vi "APC_9056_FPGA_main.vi"() -> ()   [LabVIEW 2020]
uses:
  <vilib>/Platform/TimedLoop/XDataNode/timing_clust.ctl
  <vilib>/Platform/TimedLoop/XDataNode/nitl_modes.ctl
  <vilib>/Platform/TimedLoop/XDataNode/wakeup.ctl
  <vilib>/rvi/eio/common/nirviEmuTemplateMethod_errors.vi
  <vilib>/rvi/Emulation/niFpgaGetClockAttributes.vi
  <vilib>/rvi/Emulation/niFpgaSctlEmulationGetInTimedLoop.vi
  <vilib>/rvi/Emulation/niFpgaEmulationReportErrorSimple.vi
  <vilib>/rvi/Emulation/niFpgaCriticalErrorInLSC.vi
  <vilib>/rvi/Emulation/niFpgaProcessEmulError.vi
  <vilib>/eio/EIONode/EIONode.xnode
  <vilib>/platform/TimedLoop/XDataNode/XDataNode.xnode
  <vilib>/Platform/TimedLoop/XDataNode/XDNodeRunTimeDep.lvlib
panel:
  out "counter":u32
  in  "margin":u32=250
  in  "Ticks per toggle":u32[](array[numeric])=[13000, 12000, 11000, 10000, 9000, 8000, 7000, 6000, 5000, 4000, 3000, 2000, 1000]
  out "Detected mode":i16
  out "RT counter overflow: setting SAFE mode":bool
  in  "Counter max [10 ms clock]":u32=100
  out "Watchdog counter":u32
  in  "RT watchdog":bool
  out "NI9375/DI15":bool
  out "NI9375/DI14":bool
  out "NI9375/DI13":bool
  out "NI9375/DI12":bool
  out "NI9375/DI11":bool
  out "NI9375/DI10":bool
  out "NI9375/DI9":bool
  out "NI9375/DI8":bool
  out "NI9375/DI7":bool
  out "NI9375/DI6":bool
  out "NI9375/DI5":bool
  out "NI9375/DI4":bool
  out "NI9375/DI3":bool
  out "NI9375/DI2":bool
  out "NI9375/DI1":bool
  out "NI9375/DI0":bool
  in  "NI9375/DO15":bool
  in  "NI9375/DO14":bool
  in  "NI9375/DO13":bool
  in  "NI9375/DO12":bool
  in  "NI9375/DO11":bool
  in  "NI9375/DO10":bool
  in  "NI9375/DO9":bool
  in  "NI9375/DO8":bool
  in  "NI9375/DO7":bool
  in  "NI9375/DO6":bool
  in  "NI9375/DO5":bool
  in  "NI9375/DO4":bool
  in  "NI9375/DO3":bool
  in  "NI9375/DO2":bool
  in  "NI9375/DO1":bool
  in  "NI9375/DO0":bool
  in  "NI9266/AO7":fxp<+,20,-5>
  in  "NI9266/AO6":fxp<+,20,-5>
  in  "NI9266/AO5":fxp<+,20,-5>
  in  "NI9266/AO4":fxp<+,20,-5>
  in  "NI9266/AO3":fxp<+,20,-5>
  in  "NI9266/AO2":fxp<+,20,-5>
  in  "NI9266/AO1":fxp<+,20,-5>
  in  "NI9266/AO0":fxp<+,20,-5>
  in  "NI9264/AO15":fxp<+/-,20,5>
  in  "NI9264/AO14":fxp<+/-,20,5>
  in  "NI9264/AO13":fxp<+/-,20,5>
  in  "NI9264/AO12":fxp<+/-,20,5>
  in  "NI9264/AO11":fxp<+/-,20,5>
  in  "NI9264/AO10":fxp<+/-,20,5>
  in  "NI9264/AO9":fxp<+/-,20,5>
  in  "NI9264/AO8":fxp<+/-,20,5>
  in  "NI9264/AO7":fxp<+/-,20,5>
  in  "NI9264/AO6":fxp<+/-,20,5>
  in  "NI9264/AO5":fxp<+/-,20,5>
  in  "NI9264/AO4":fxp<+/-,20,5>
  in  "NI9264/AO3":fxp<+/-,20,5>
  in  "NI9264/AO2":fxp<+/-,20,5>
  in  "NI9264/AO1":fxp<+/-,20,5>
  in  "NI9264/AO0":fxp<+/-,20,5>
  out "dT HB (ms)":u32
  out "dT inj (ticks)":u32
  out "FPGA Hearbeat":bool
  out "Chassis Temp Raw (x4 C)":i16=143
  # "This is low level FPGA interface only! \nDO NOT USE DIRECTLY\nUse RT module to configure"
  # "NI9264 interface"
  # "General Monitoring & Control"
  # "NI9266 interface"
  # "USER LED1 is also \nbroadcasting the \nhearbeat at 1Hz"
  # "NI9375 interface"
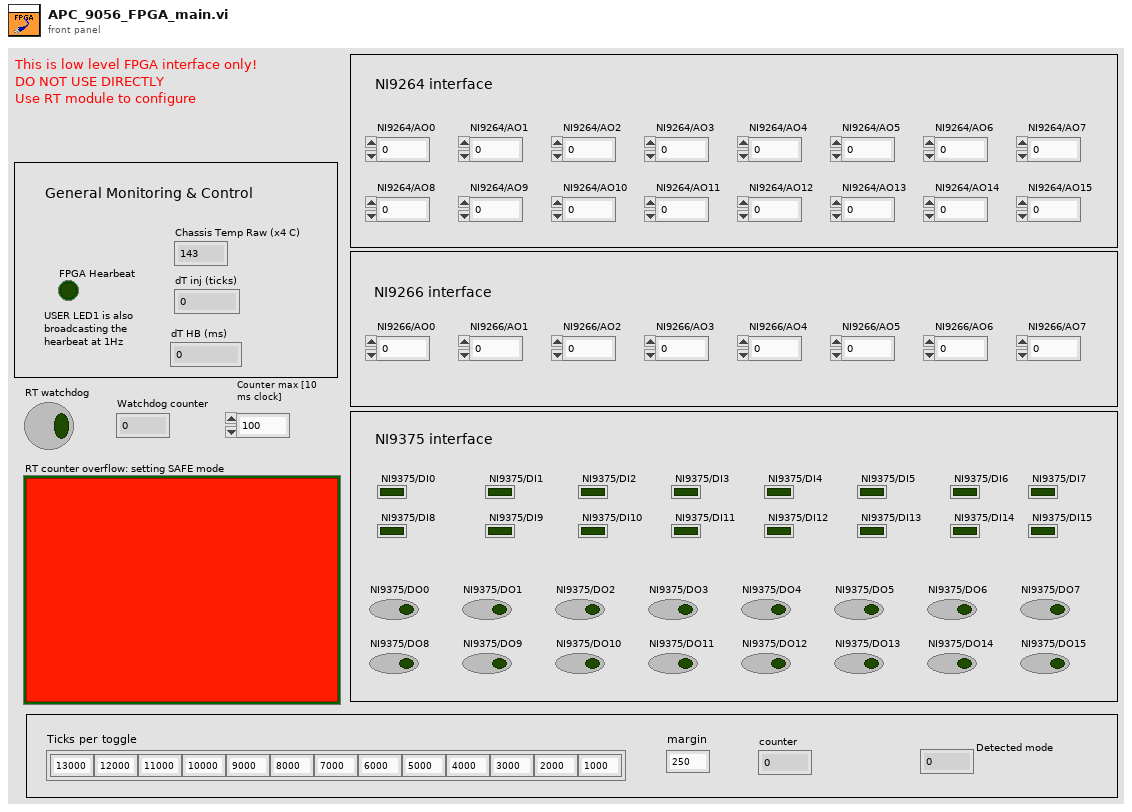
[diagram p1: front panel]
types:
  T1 = typedef "XDNodeRunTimeDep.lvlib/timing_clust.ctl" = cluster{"Expected End [f-1]":u64, "Actual End [f-1]":u64, "Finished Late? [f-1]":bool, "Expected End [i-1]":u64, "Actual End [i-1]":u64, "Finished Late? [i-1]":bool, "Expected Start [i]":u64, "Actual Start [i]":u64, "Expected Start [f]":u64, "Actual Start [f]":u64, "Source Name":string, "Structure Name":string, "Period":i64, "Deadline":i64, "Offset":i64, "Start":i64, "Priority":i32, "Timeout":i32, "Mode":T2, "Wakeup Reason":T3, "Error":errorcluster, "Source Type":string, "Secondary Source Type":string, "Global End Time":u64, "Global Start Time":u64, "Frame Duration":u64, "Iteration Duration":u64, "Assigned CPU":i32, "I/O Scan Engine Mode":u32}
  T2 = typedef "XDNodeRunTimeDep.lvlib/nitl_modes.ctl" = enum32{"No Change", "Process missed periods, maintain original phase", "Discard missed periods, maintain original phase", "Process missed periods, ignore original phase", "Discard missed periods, ignore original phase"}
  T3 = typedef "XDNodeRunTimeDep.lvlib/wakeup.ctl" = enum32{"Normal", "Aborted", "Asynchronous wakeup", "Timing source error", "Timed loop error", "Timeout"}
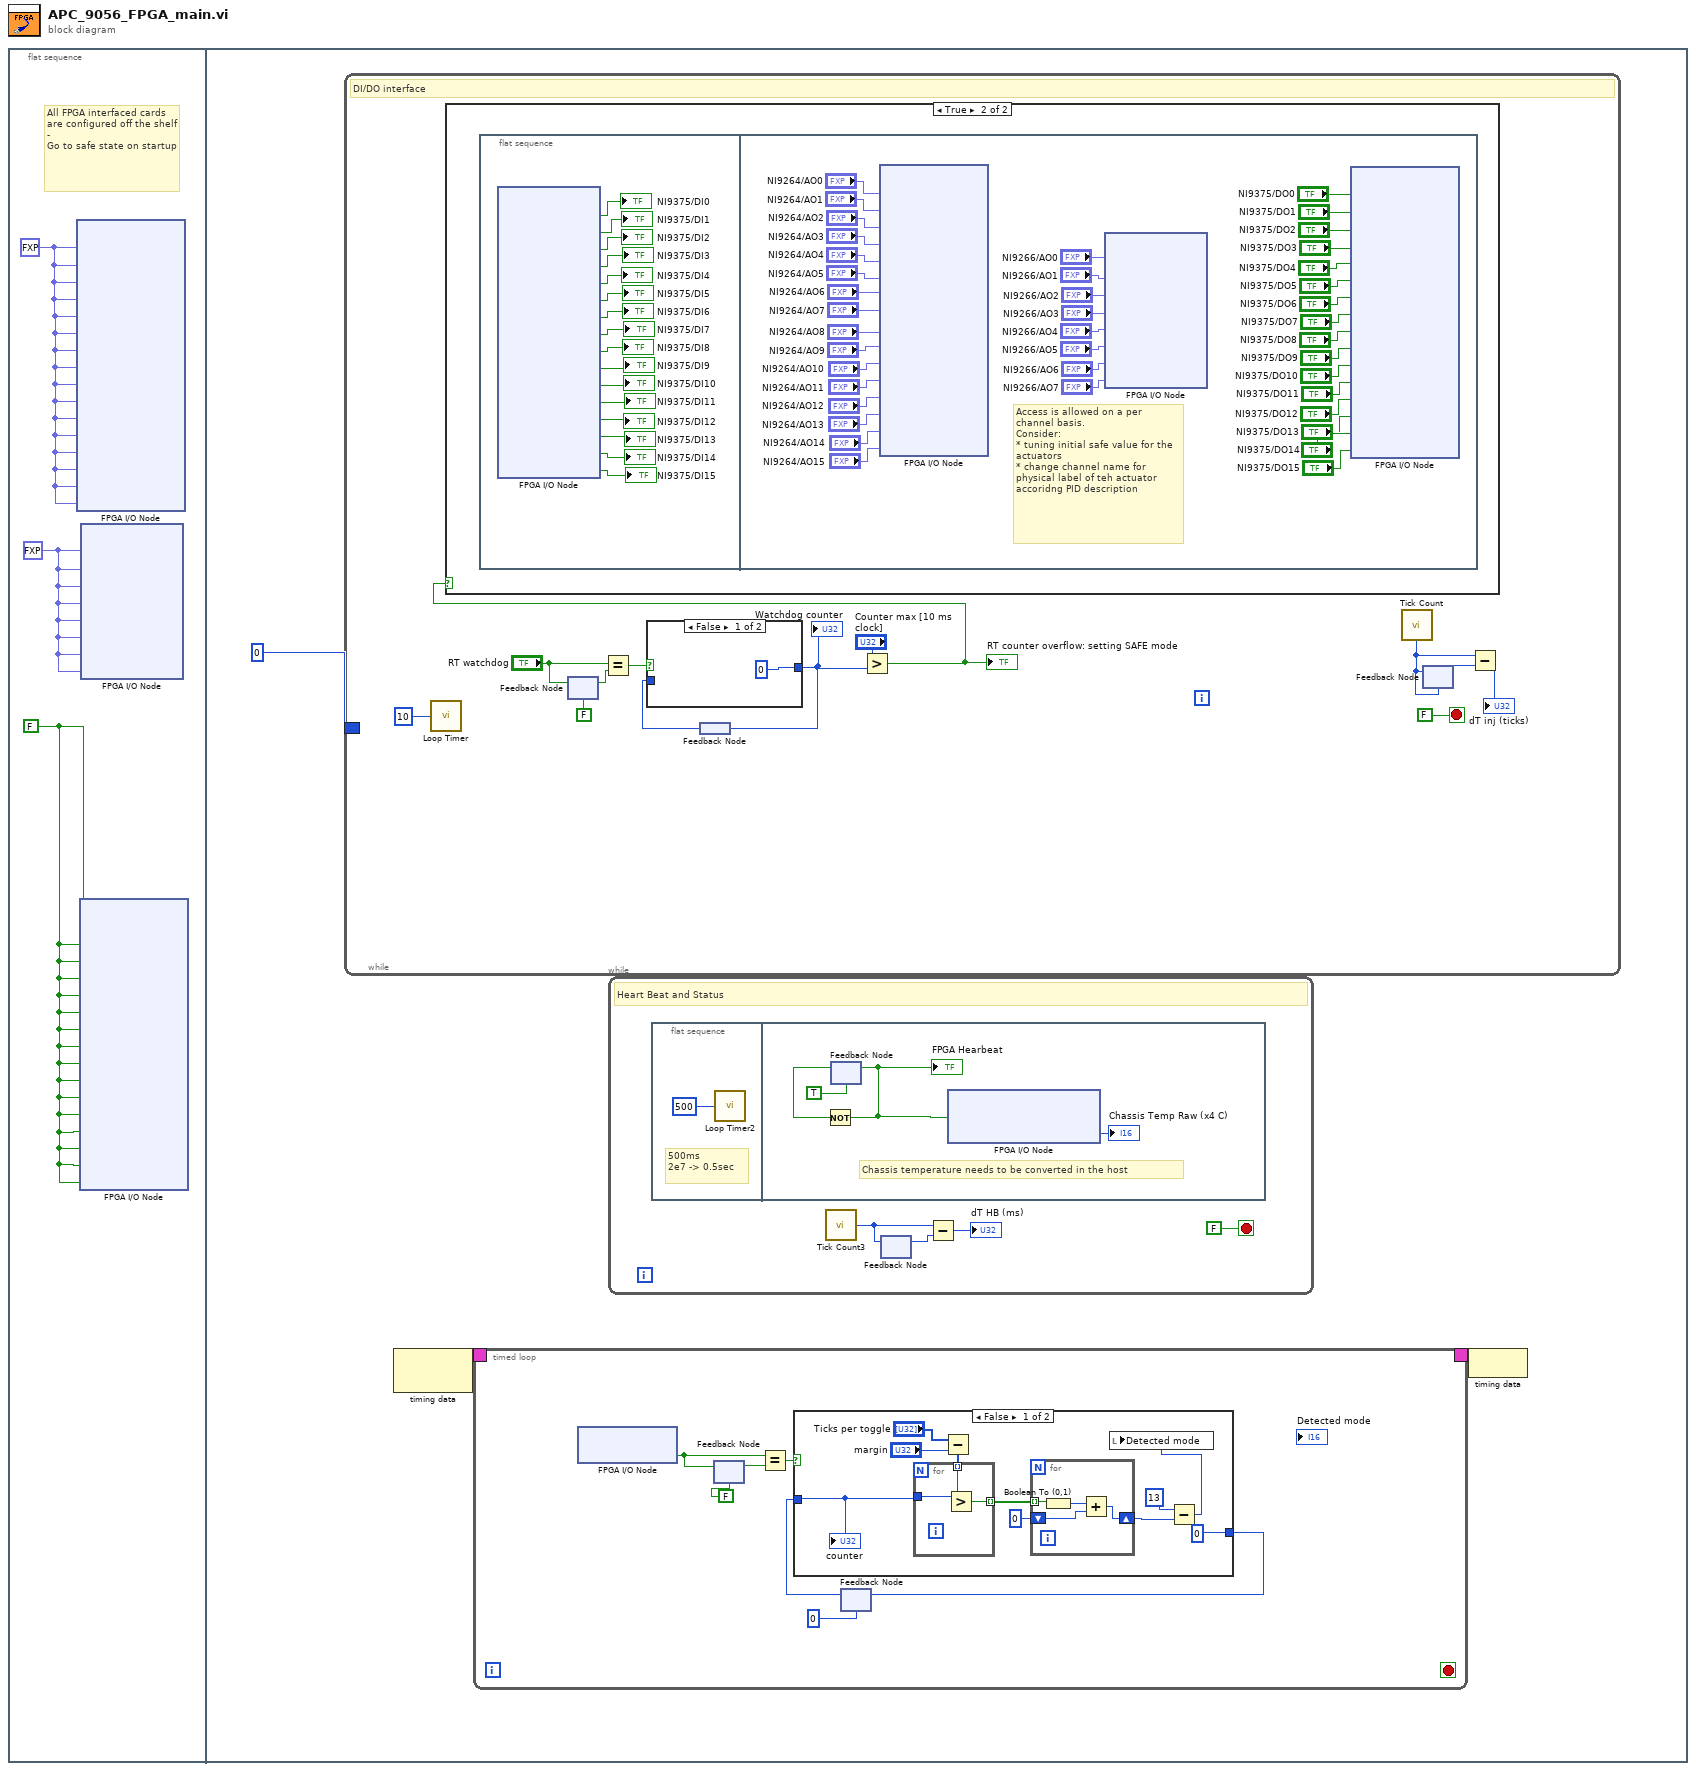
[diagram p0: block diagram]
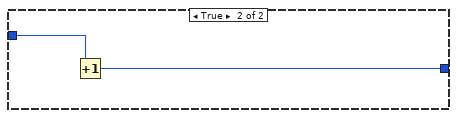
[diagram p2: hidden frame]
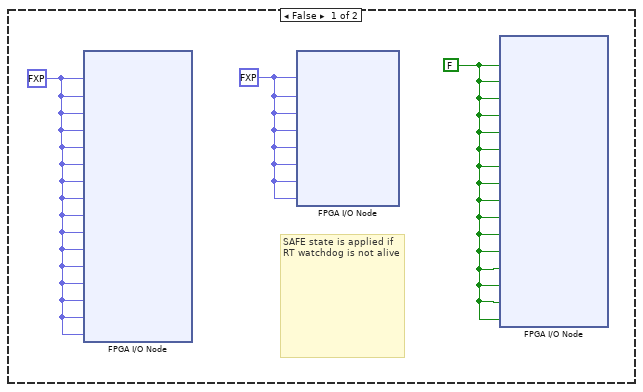
[diagram p3: hidden frame]
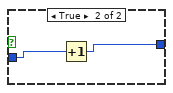
[diagram p4: hidden frame]
diagram:
  n1 = flat-sequence {
    frame #0 {
      w1 = FALSE ("Mod1/DO0")
      w2 = fxp<+,20,-5> 0.0 ("Mod3/AO0")
      w3 = fxp<+/-,20,5> 0.0 ("Mod2/AO0")
      # "All FPGA interfaced cards are configured off the shelf\n-\nGo to safe state on startup"
      n2 = xnode ("FPGA I/O Node")("Mod2/AO0"=w3, "Mod2/AO1"=w3, "Mod2/AO2"=w3, "Mod2/AO3"=w3, "Mod2/AO4"=w3, "Mod2/AO5"=w3, "Mod2/AO6"=w3, "Mod2/AO7"=w3, "Mod2/AO8"=w3, "Mod2/AO9"=w3, "Mod2/AO10"=w3, "Mod2/AO11"=w3, "Mod2/AO12"=w3, "Mod2/AO13"=w3, "Mod2/AO14"=w3, "Mod2/AO15"=w3) -> ()  [unwired: 16 in, 16 out]
      n3 = xnode "FPGA I/O Node"("Mod1/DO0"=w1, "Mod1/DO1"=w1, "Mod1/DO2"=w1, "Mod1/DO3"=w1, "Mod1/DO4"=w1, "Mod1/DO5"=w1, "Mod1/DO6"=w1, "Mod1/DO7"=w1, "Mod1/DO8"=w1, "Mod1/DO9"=w1, "Mod1/DO10"=w1, "Mod1/DO11"=w1, "Mod1/DO12"=w1, "Mod1/DO13"=w1, "Mod1/DO14"=w1, "Mod1/DO15"=w1) -> ()  [unwired: 16 in, 16 out]
      n4 = xnode "FPGA I/O Node"("Mod3/AO0"=w2, "Mod3/AO1"=w2, "Mod3/AO2"=w2, "Mod3/AO3"=w2, "Mod3/AO4"=w2, "Mod3/AO5"=w2, "Mod3/AO6"=w2, "Mod3/AO7"=w2) -> ()  [unwired: 8 in, 8 out]
    }
    frame #1 {
      n5 = while {
        border: 0 -> [_]
        stop <- FALSE stop-if-true
        # "DI/DO interface"
        n6 = call "Loop Timer"("Count(mSec)"=u32 10) -> ()  [unwired: 1 out]
        n7 = feedback #1(FALSE ("RT watchdog")) -> (w43:bool)
        n8 = feedback-in #1("RT watchdog") -> ()
        n9 = Equal?(x="RT watchdog", y=w43) -> (x = y?=w42:bool)
        n10 = feedback #2() -> (w41:u32)
        n11 = case shown="False" w42 {
          tunnel: [u32 0 w110] -> w40
          tunnel: w41 -> [_ w111]
          frame False {
          }
          frame True {
            n12 = Increment(x=w111) -> (x+1=w110:u32)
          }
        }
        "Watchdog counter" <- w40
        n13 = feedback-in #2(w40) -> ()
        n14 = Greater?(x="Counter max [10 ms clock]", y=w40) -> (0:w38:bool)
        "RT counter overflow: setting SAFE mode" <- w38
        n15 = case shown="True" w38 {
          frame False {
            w50 = FALSE ("Mod1/DO0")
            w51 = fxp<+,20,-5> 0.0 ("Mod3/AO0")
            w52 = fxp<+/-,20,5> 0.0 ("Mod2/AO0")
            # "SAFE state is applied if RT watchdog is not alive"
            n16 = xnode ("FPGA I/O Node")("Mod2/AO0"=w52, "Mod2/AO1"=w52, "Mod2/AO2"=w52, "Mod2/AO3"=w52, "Mod2/AO4"=w52, "Mod2/AO5"=w52, "Mod2/AO6"=w52, "Mod2/AO7"=w52, "Mod2/AO8"=w52, "Mod2/AO9"=w52, "Mod2/AO10"=w52, "Mod2/AO11"=w52, "Mod2/AO12"=w52, "Mod2/AO13"=w52, "Mod2/AO14"=w52, "Mod2/AO15"=w52) -> ()  [unwired: 16 in, 16 out]
            n17 = xnode "FPGA I/O Node"("Mod3/AO0"=w51, "Mod3/AO1"=w51, "Mod3/AO2"=w51, "Mod3/AO3"=w51, "Mod3/AO4"=w51, "Mod3/AO5"=w51, "Mod3/AO6"=w51, "Mod3/AO7"=w51) -> ()  [unwired: 8 in, 8 out]
            n18 = xnode "FPGA I/O Node"("Mod1/DO0"=w50, "Mod1/DO1"=w50, "Mod1/DO2"=w50, "Mod1/DO3"=w50, "Mod1/DO4"=w50, "Mod1/DO5"=w50, "Mod1/DO6"=w50, "Mod1/DO7"=w50, "Mod1/DO8"=w50, "Mod1/DO9"=w50, "Mod1/DO10"=w50, "Mod1/DO11"=w50, "Mod1/DO12"=w50, "Mod1/DO13"=w50, "Mod1/DO14"=w50, "Mod1/DO15"=w50) -> ()  [unwired: 16 in, 16 out]
          }
          frame True {
            n19 = flat-sequence {
              frame #0 {
                n20 = xnode "FPGA I/O Node"() -> ("Mod1/DI0"=→"NI9375/DI0":bool, "Mod1/DI1"=→"NI9375/DI1":bool, "Mod1/DI2"=→"NI9375/DI2":bool, "Mod1/DI3"=→"NI9375/DI3":bool, "Mod1/DI4"=→"NI9375/DI4":bool, "Mod1/DI5"=→"NI9375/DI5":bool, "Mod1/DI6"=→"NI9375/DI6":bool, "Mod1/DI7"=→"NI9375/DI7":bool, "Mod1/DI8"=→"NI9375/DI8":bool, "Mod1/DI9"=→"NI9375/DI9":bool, "Mod1/DI10"=→"NI9375/DI10":bool, "Mod1/DI11"=→"NI9375/DI11":bool, "Mod1/DI12"=→"NI9375/DI12":bool, "Mod1/DI13"=→"NI9375/DI13":bool, "Mod1/DI14"=→"NI9375/DI14":bool, "Mod1/DI15"=→"NI9375/DI15":bool)  [unwired: 16 in, 16 out]
              }
              frame #1 {
                # "Access is allowed on a per channel basis.\nConsider: \n* tuning initial safe value for the actuators\n* change channel name for physical label of teh actuator accoridng PID description"
                n21 = xnode ("FPGA I/O Node")("Mod2/AO0"="NI9264/AO0", "Mod2/AO1"="NI9264/AO1", "Mod2/AO2"="NI9264/AO2", "Mod2/AO3"="NI9264/AO3", "Mod2/AO4"="NI9264/AO4", "Mod2/AO5"="NI9264/AO5", "Mod2/AO6"="NI9264/AO6", "Mod2/AO7"="NI9264/AO7", "Mod2/AO8"="NI9264/AO8", "Mod2/AO9"="NI9264/AO9", "Mod2/AO10"="NI9264/AO10", "Mod2/AO11"="NI9264/AO11", "Mod2/AO12"="NI9264/AO12", "Mod2/AO13"="NI9264/AO13", "Mod2/AO14"="NI9264/AO14", "Mod2/AO15"="NI9264/AO15") -> ()  [unwired: 16 in, 16 out]
                n22 = xnode "FPGA I/O Node"("Mod3/AO0"="NI9266/AO0", "Mod3/AO1"="NI9266/AO1", "Mod3/AO2"="NI9266/AO2", "Mod3/AO3"="NI9266/AO3", "Mod3/AO4"="NI9266/AO4", "Mod3/AO5"="NI9266/AO5", "Mod3/AO6"="NI9266/AO6", "Mod3/AO7"="NI9266/AO7") -> ()  [unwired: 8 in, 8 out]
                n23 = xnode "FPGA I/O Node"("Mod1/DO0"="NI9375/DO0", "Mod1/DO1"="NI9375/DO1", "Mod1/DO2"="NI9375/DO2", "Mod1/DO3"="NI9375/DO3", "Mod1/DO4"="NI9375/DO4", "Mod1/DO5"="NI9375/DO5", "Mod1/DO6"="NI9375/DO6", "Mod1/DO7"="NI9375/DO7", "Mod1/DO8"="NI9375/DO8", "Mod1/DO9"="NI9375/DO9", "Mod1/DO10"="NI9375/DO10", "Mod1/DO11"="NI9375/DO11", "Mod1/DO12"="NI9375/DO12", "Mod1/DO13"="NI9375/DO13", "Mod1/DO14"="NI9375/DO14", "Mod1/DO15"="NI9375/DO15") -> ()  [unwired: 16 in, 16 out]
              }
            }
          }
        }
        n24 = call "Tick Count"() -> ("Tick Count(Ticks)"=w48:u32)
        n25 = feedback-in #3(w48) -> ()
        n26 = feedback #3(w48) -> (w49:u32)
        n27 = Subtract(x=w48, y=w49) -> (x-y=→"dT inj (ticks)":u32)
      }
      n28 = node-c288() -> (w5:T1)  [unwired: 1 in]
      n29 = timed-loop {
        timing: w5 -> [_]
        timing-out: [_] -> w4
        stop <- _ stop-if-true
        n30 = xnode ("FPGA I/O Node")() -> ("cRIO_Trig7"=w8:bool)  [unwired: 1 in, 1 out]
        n31 = feedback #4(FALSE ("cRIO_Trig7")) -> (w7:bool)
        n32 = feedback-in #4(w8) -> ()
        n33 = Equal?(x=w8, y=w7) -> (x = y?=w9:bool)
        n34 = feedback #5(u32 0) -> (w13:u32)
        n35 = case shown="False" w9 {
          tunnel: [u32 0 w32] -> w12
          tunnel: w13 -> [w22 w31]
          frame False {
            n36 = Subtract(x="Ticks per toggle", y="margin") -> (x-y=w19:u32[])
            n37 = for {
              tunnel: w22 -> [w30]
              tunnel: w19 -> [w29] mode=indexing
              tunnel: [w28] -> w18 mode=indexing
              n38 = Greater?(x=w30, y=w29) -> (0:w28:bool)
            }
            n39 = for {
              tunnel: w18 -> [w27] mode=indexing
              shift-right: [w25] -> w16
              shift-left: i16 0 -> [w24]
              n40 = Boolean To (0,1)(Boolean=w27) -> (0, 1=w26:i16)
              n41 = Add(x=w26, y=w24) -> (x+y=w25:i16)
            }
            n42 = Subtract(x=i16 13, y=w16) -> (x-y=w14:i16)
            n43 = local write "Detected mode"(w14) -> ()
            "counter" <- w22
          }
          frame True {
            n44 = Increment(x=w31) -> (x+1=w32:u32)
          }
        }
        n45 = feedback-in #5(w12) -> ()
      }
      n46 = while {
        stop <- FALSE stop-if-true
        # "Heart Beat and Status"
        n47 = flat-sequence {
          frame #0 {
            # "500ms\n2e7 -> 0.5sec"
            n48 = call "Loop Timer2"("Count(mSec)"=u32 500) -> ()  [unwired: 1 out]
          }
          frame #1 {
            # "Chassis temperature needs to be converted in the host"
            n49 = feedback #6(TRUE ("USER FPGA LED")) -> (w118:bool)
            n50 = Not(x=w118) -> (.not. x?=w117:bool)
            "FPGA Hearbeat" <- w117
            n51 = feedback-in #6(w117) -> ()
            n52 = xnode "FPGA I/O Node"("USER FPGA LED"=w117) -> ("Chassis Temperature"=→"Chassis Temp Raw (x4 C)":i16)  [unwired: 2 in, 2 out]
          }
        }
        n53 = call "Tick Count3"() -> ("Tick Count(mSec)"=w114:u32)
        n54 = feedback #7() -> (w115:u32)  [unwired: 1 in]
        n55 = feedback-in #7(w114) -> ()
        n56 = Subtract(x=w114, y=w115) -> (x-y=→"dT HB (ms)":u32)
      }
      n57 = node-c288(w4) -> ()
    }
  }
